vi "Simple Function (SubVI).vi"(11 "f(x) (mm -> deg)":string) -> (0 "Stage Position (mm)":dbl, 2 "Next Angle (deg)":dbl)   [LabVIEW 2012]
uses:
  variables/GlobalUI.vi
  Rotation Mount Global.vi
  <vilib>/gmath/NI_Gmath.lvlib
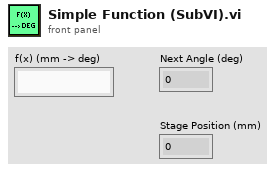
[diagram p1: front panel]
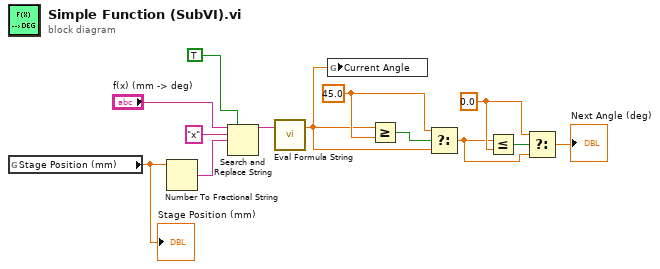
[diagram p0: block diagram]
diagram:
  w4 = 0.0 ("y")
  w6 = 45.0 ("y")
  n1 = global read "GlobalUI.vi" "Stage Position (mm)"() -> (w13:dbl)
  "Stage Position (mm)" <- w13
  n2 = Number To Fractional String(number=w13) -> (F-format string=w11:string)  [unwired: 3 in]
  n3 = Search and Replace String(replace all?=TRUE ("replace all? (F)"), input string="f(x) (mm -> deg)", search string="x", replace string=w11) -> (result string=w12:string)  [unwired: 4 in, 3 out]
  n4 = call <vilib>:"Eval Formula String.vi"("formula"=w12) -> ("y value"=w3:dbl)  [unwired: 1 in, 1 out]
  n5 = global write "Rotation Mount Global.vi" "Current Angle"(w3) -> ()
  n6 = Greater Or Equal?(x=w3, y=w6) -> (x >= y?=w7:bool)
  n7 = Select(t=w6, s=w7, f=w3) -> (s? t:f=w1:dbl)
  n8 = Less Or Equal?(x=w1, y=w4) -> (x <= y?=w5:bool)
  n9 = Select(t=w4, s=w5, f=w1) -> (s? t:f=→"Next Angle (deg)":dbl)
